vi "LEBITplc.CreateLogFile.vi"(0 "i ref in":refnum<vi>, 1 "File Name":string, 2 "i attribute in":T1, 3 "nickName":string, 4 "value\nnobase":dbl, 5 "error in":errorcluster, 7 "Enum":enum16{"Set Value", "Loaded File"}(ring)=enum."Loaded File", 9 "LoadOrSave":string="Load ") -> (14 "i ref out":refnum<vi>, 16 "i attribute out":T1, 19 "error out":errorcluster)   [LabVIEW 2014, in "LEBITplc.lvlib"]
uses:
  LEBITplc.lvlib
  LEBITplc.i attribute.ctl
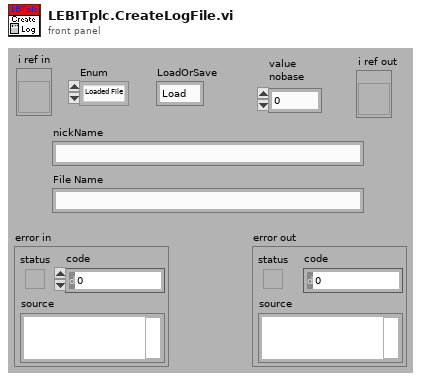
[diagram p1: front panel]
types:
  T1 = typedef "LEBITplc.lvlib/LEBITplc.i attribute.ctl" = cluster{"LLFLocation":string, "SetFileLocation":string, "nickNames":string[], "setValuePLCServiceID":i32[], "GUIServiceID":i32[], "monValuePLC":string[], "SetValueServiceID":i32[], "MonValueServiceID":i32[], "SetValue":dbl[][], "SetValueMin":dbl[], "SetValueMax":dbl[], "SetValueInfoServiceID":i32[], "GUINames":string[], "ListOfBases":string[], "Scale":dbl[], "Offset":dbl[], "setValuePLC":string[], "BaseName":string[], "ScaleServiceID":i32[], "OffsetServiceID":i32[], "AllPLCValues":string[], "CondSpecialArray":string[][], "CondSpecialIndex":i32[], "CondSpecialMonValue":dbl[], "RecentlyChanged":i32[], "SetFileLocationID":i32, "Dependent-Monitors":string[][], "LastLoadedFiles":string[], "IonGuideCalibLocation":string, "Monitor Dependent":string[], "Special":string[], "PLC?":bool[], "Start Date":string, "ListOfBasesServiceID":i32, "SETRA VISA resource":refnum<visa-resource-name>}
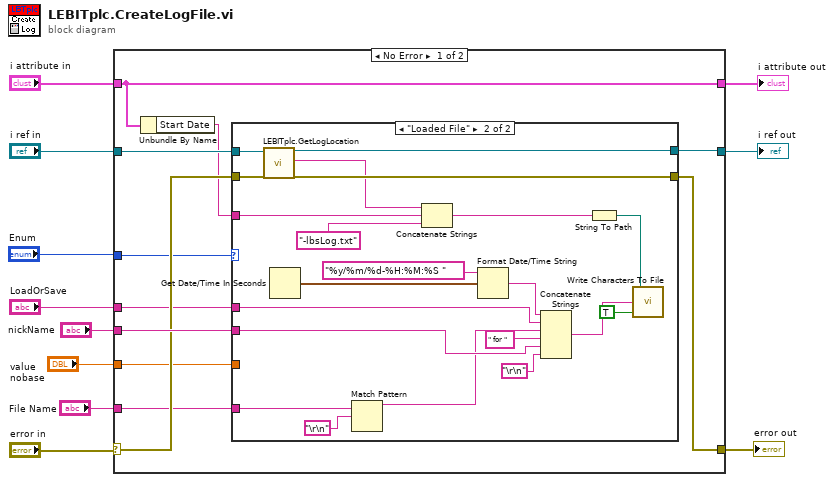
[diagram p0: block diagram]
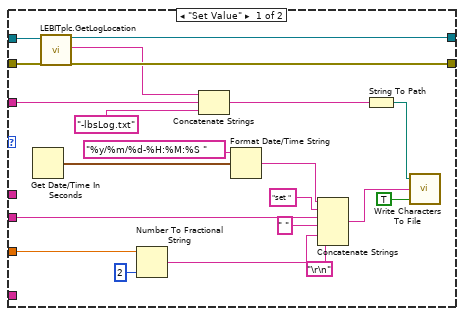
[diagram p2: hidden frame]
diagram:
  n1 = case shown="No Error" "error in" {
    selector: "error in" -> [w19 w67]
    tunnel: "nickName" -> [w22 _]
    tunnel: [w18 w67] -> w9
    tunnel: "i ref in" -> [w21 w66]
    tunnel: [w20 w66] -> w5
    tunnel: "i attribute in" -> [w14 w65]
    tunnel: [w14 w65] -> w7
    tunnel: "value\nnobase" -> [w17 _]
    tunnel: "Enum" -> [w16 _]
    tunnel: "File Name" -> [w15 _]
    tunnel: "LoadOrSave" -> [w12 _]
    frame No Error {
      n2 = Unbundle By Name(w14) -> ("Start Date"=w13:string)
      n3 = case shown="\"Loaded File\"" w16 {
        tunnel: w22 -> [w27 w53]
        tunnel: w21 -> [w36 w58]
        tunnel: [w35 w57] -> w20
        tunnel: w19 -> [w34 w56]
        tunnel: [w33 w55] -> w18
        tunnel: w17 -> [w29 _]
        tunnel: w15 -> [_ w51]
        tunnel: w13 -> [w24 w45]
        tunnel: w12 -> [_ w44]
        frame "Set Value" {
          n4 = Get Date/Time In Seconds() -> (seconds since 1Jan1904=w26:timestamp)
          n5 = call "LEBITplc.GetLogLocation.vi"("i ref in"=w36, "error in (no error)"=w34) -> ("i ref out"=w35:refnum<vi>, "log location"=w32:string, "error out 2"=w33:errorcluster)  [unwired: 15 in]
          n6 = Number To Fractional String(number=w29, precision (6)=i16 2) -> (F-format string=w30:string)  [unwired: 2 in]
          n7 = Concatenate Strings(w32, w24, "-lbsLog.txt" ("time format string (%c)")) -> (w37:string)
          n8 = Format Date/Time String(time format string (%c)="%y/%m/%d-%H:%M:%S ", seconds (now)=w26) -> (date/time string=w23:string)  [unwired: 1 in]
          n9 = Concatenate Strings(w23, "set ", w27, " " ("string"), w30, "\r\n") -> (w41:string)
          n10 = String To Path(string=w37) -> (path=w43:path)
          n11 = call <vilib>:"Write Characters To File.vi"("append to file? (new file:F)"=TRUE, "character string"=w41, "file path (dialog if empty)"=w43) -> ()  [unwired: 2 in, 1 out]
        }
        frame "Loaded File" {
          n12 = call "LEBITplc.GetLogLocation.vi"("i ref in"=w58, "error in (no error)"=w56) -> ("i ref out"=w57:refnum<vi>, "log location"=w54:string, "error out 2"=w55:errorcluster)  [unwired: 15 in]
          n13 = Get Date/Time In Seconds() -> (seconds since 1Jan1904=w49:timestamp)
          n14 = Match Pattern(string=w51, regular expression="\r\n") -> (before substring=w50:string)  [unwired: 1 in, 3 out]
          n15 = Concatenate Strings(w54, w45, "-lbsLog.txt" ("time format string (%c)")) -> (w59:string)
          n16 = Format Date/Time String(time format string (%c)="%y/%m/%d-%H:%M:%S ", seconds (now)=w49) -> (date/time string=w47:string)  [unwired: 1 in]
          n17 = Concatenate Strings(w47, w44, w50, " for " ("string"), w53, "\r\n") -> (w62:string)
          n18 = String To Path(string=w59) -> (path=w64:path)
          n19 = call <vilib>:"Write Characters To File.vi"("append to file? (new file:F)"=TRUE, "character string"=w62, "file path (dialog if empty)"=w64) -> ()  [unwired: 2 in, 1 out]
        }
      }
    }
    frame Error {
    }
  }
  "error out" <- w9
  "i ref out" <- w5
  "i attribute out" <- w7
